vi "Get Default Value.vi"(8 "error in (no error)":errorcluster, 11 "Item Ref in":T1 format="%.0x") -> (0 "error out":errorcluster, 2 "DefaultValue":dbl, 3 "Item Ref out":T1)   [LabVIEW 2013, in "PWM System Explorer.lvlib"]
uses:
  PWM System Explorer.lvlib
  <vilib>/NI Veristand/Custom Device API/Custom Device Item Ref.ctl
  NationalInstruments.VeriStand.SystemDefinitionAPI
  <vilib>/NI Veristand/Custom Device Offline API/Custom Device Offline API.lvlib
  <vilib>/NI Veristand/Custom Device API/Custom Device API.lvlib
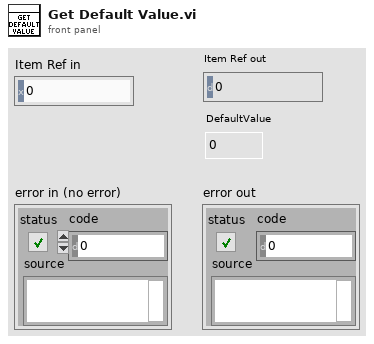
[diagram p1: front panel]
types:
  T1 = typedef "Custom Device API.lvlib/Custom Device Item Ref.ctl" = u64
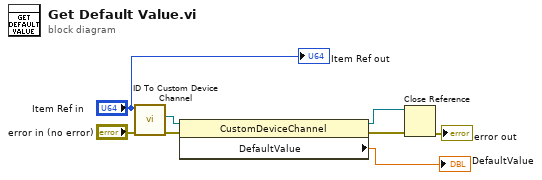
[diagram p0: block diagram]
diagram:
  n1 = call <vilib>:"ID To Custom Device Channel.vi"("error in (no error)"="error in (no error)", "ID in"="Item Ref in") -> ("error out"=w3:errorcluster, "Channel"=w4:refnum<k24>)  [unwired: 7 in, 1 out]
  n2 = property class="CustomDeviceChannel"(reference=w4, error in=w3) -> (reference out=w7:refnum<k24>, error out=w5:errorcluster, "DefaultValue"=→"DefaultValue":dbl)
  n3 = Close Reference(reference=w7, error in (no error)=w5) -> (error out=→"error out":errorcluster)
  "Item Ref out" <- "Item Ref in"
